vi "List Files.vi"(8 "error in (no error)":errorcluster, 9 "depth":i32=-1, 10 "ģʽ":string, 11 "stripped path":path) -> (0 "error out":errorcluster, 3 "files":path[](array[path]))   [LabVIEW 2015]
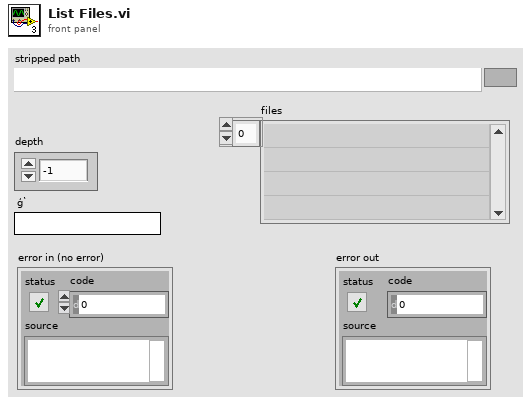
[diagram p1: front panel]
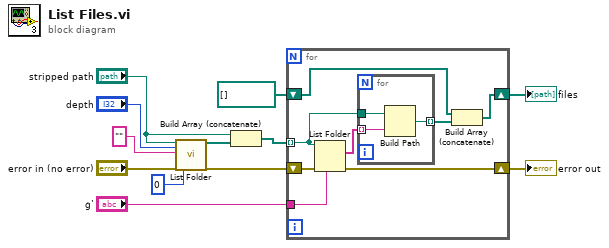
[diagram p0: block diagram]
diagram:
  n1 = call "List Folder.vi"("stripped path"="stripped path", "depth"="depth", "ģʽ"="", "error in (no error)"="error in (no error)", "depth index"=0) -> ("files"=w7:path[], "error out"=w10:errorcluster)  [unwired: 13 in]
  n2 = Build Array (concatenate)("stripped path", w7) -> (w2:path[])
  n3 = for {
    tunnel: "ģʽ" -> [w20]
    tunnel: w2 -> [w17] mode=indexing
    shift-right: [w18] -> w9
    shift-left: w10 -> [w19]
    shift-right: [w14] -> w6
    shift-left: path[] [] -> [w13]
    n4 = List Folder(path=w17, pattern=w20, error in=w19) -> (filenames=w16:string[], error out=w18:errorcluster)  [unwired: 1 in, 2 out]
    n5 = for {
      tunnel: w17 -> [w23]
      tunnel: w16 -> [w22] mode=indexing
      tunnel: [w21] -> w15 mode=indexing
      n6 = Build Path(base path=w23, name or relative path=w22) -> (appended path=w21:path)
    }
    n7 = Build Array (concatenate)(w13, w15) -> (w14:path[])
  }
  "files" <- w6
  "error out" <- w9
